vi "Test Create and Add Instrument2.vi"(11 "Test Case In":refnum<class "Measure and Stimulus Subsystems.lvclass">) -> (0 "error out":errorcluster, 3 "Test Case Out":refnum<class "Measure and Stimulus Subsystems.lvclass">)   [LabVIEW 2023, in "Measure and Stimulus Subsystems.lvclass"]
uses:
  Measure and Stimulus Subsystems.lvclass
  C:/Program Files/National Instruments/LabVIEW 2023/vi.lib/Astemes/LUnit/Test Case.lvclass
  Measure and Stimulus Subsystems/Measure and Stimulus Subsystems.lvclass
  Measure and Stimulus Subsystems/Measure and Stimulus Subsystems.lvclass/Measure and Stimulus Subsystems.ctl
  <vilib>/Astemes/LUnit/Test Case.lvclass/Test Case.ctl
  4993e8ee-a06a-463a-9684-69129f64d5ce.vi
  <vilib>/Astemes/LUnit/Append Pass Result.vi
  <vilib>/Astemes/LUnit/Append Fail Result.vi
  <vilib>/Astemes/LUnit/Describe Comparison.vi
  <vilib>/Astemes/LUnit/Compare Variants.vi
  <vilib>/Astemes/LUnit/Run In UI.vi
  <vilib>/Utility/error.llb/Clear Errors.vi
  Instrument/utils/Instrument_GetAttributes.vi
  <vilib>/Astemes/LUnit/Describe Variant.vi
  Interfaces/IConfigure/IConfigure.lvclass
  Instrument/Instrument.lvclass
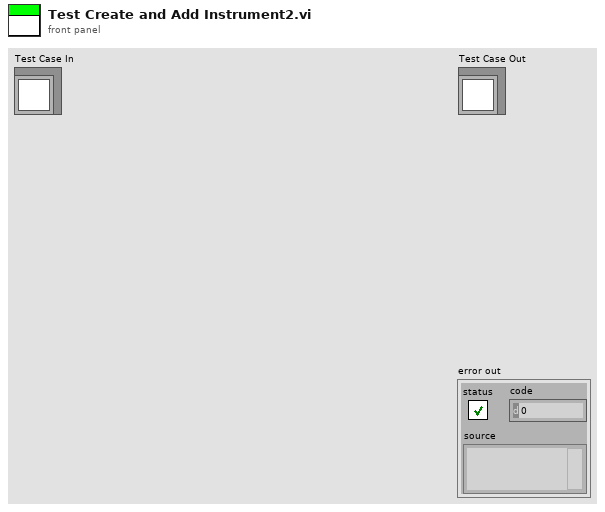
[diagram p1: front panel]
types:
  T1 = map{string, cluster{"Instrument":refnum<class "Instrument.lvclass">, "Ref Count":u8}}
  T2 = cluster{"Instrument":refnum<class "Instrument.lvclass">, "Ref Count":u8}
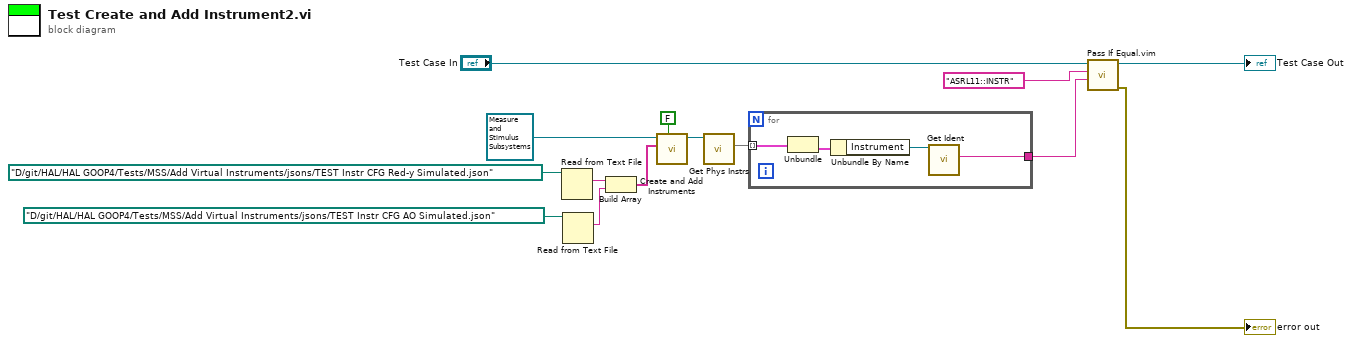
[diagram p0: block diagram]
diagram:
  n1 = Read from Text File(file (use dialog)=path "D:/git/HAL/HAL GOOP4/Tests/MSS/Add Virtual Instruments/jsons/TEST Instr CFG Red-y Simulated.json") -> (text=w8:string)  [unwired: 3 in, 3 out]
  n2 = Read from Text File(file (use dialog)=path "D:/git/HAL/HAL GOOP4/Tests/MSS/Add Virtual Instruments/jsons/TEST Instr CFG AO Simulated.json") -> (text=w5:string)  [unwired: 3 in, 3 out]
  n3 = Build Array(w8, w5) -> (w7:string[])
  n4 = call "Create and Add Instruments.vi"("Is Target?"=FALSE, "Physical Intr CFGs"=w7, "MSS in"=refnum<class "Measure and Stimulus Subsystems.lvclass"> refnum) -> ("MSS out"=w4:refnum<class "Measure and Stimulus Subsystems.lvclass">)  [unwired: 6 in, 2 out]
  n5 = call "Get Phys Instrs.vi"("MSS in"=w4) -> ("Phys Instr"=w3:T1)  [unwired: 9 in, 1 out]
  n6 = for {
    tunnel: w3 -> [w18] mode=indexing
    tunnel: [w15] -> w2
    n7 = Unbundle(w18) -> ("Phys Instr"=w17:T2)  [unwired: 1 out]
    n8 = Unbundle By Name(w17) -> ("Instrument"=w16:refnum<class "Instrument.lvclass">)
    n9 = call "Get Ident.vi"("reference in"=w16) -> ("Instr Ident"=w15:string)  [unwired: 8 in, 2 out]
  }
  n10 = call "Pass If Equal.vim"("Actual"=w2, "Expected"="ASRL11::INSTR", "LUnit Test Case In"="Test Case In") -> ("error out"=→"error out":errorcluster, "LUnit Test Case Out"=→"Test Case Out":refnum<class "Measure and Stimulus Subsystems.lvclass">)  [unwired: 7 in]
